vi "PH_SSAC.ProcCases.vi"(0 "i ref in":refnum<vi>, 1 "selector":string, 2 "Data":T1, 3 "call cluster":T2={"Object"="", "Selector"="", "CallType"=enum."synchronous", "Async Object"="", "Async Selector"="", "Data Descriptor"="", "Data"=[], "Error #"=0, "Expire"=0}, 5 "error in (no error)":errorcluster) -> (14 "i ref out":refnum<vi>, 17 "answer cluster":T2={"Object"="", "Selector"="", "CallType"=enum."synchronous", "Async Object"="", "Async Selector"="", "Data Descriptor"="", "Data"=[], "Error #"=0, "Expire"=0}, 19 "error out":errorcluster)   [LabVIEW 2014, in "PH_SSAC.lvlib"]
doc: "This method is called by a process from within the default case in the event loop. The methods of a class that are linked to events will be called from THIS method. Add your code here."
uses:
  PH_SSAC.lvlib
  CS_Core/CSSystem/CoreDefs/CoreDefs.call_type.ctl
  CS_Core/BaseProcess/BaseProcess.descriptor string definition.ctl
  CS_Core/CSSystem/CoreDefs/CoreDefs.rawDataType.ctl
  CS_Core/CSSystem/CoreLib/CoreLib.string 2 byte array.vi
  CS_Core/CSSystem/CoreLib/CoreLib.byte array 2 int.vi
  CS_Core/CSSystem/CoreLib/CoreLib.byte array 2 short.vi
  CS_Core/CSSystem/CoreLib/CoreLib.byte array 2 double.vi
  CS_Core/BaseProcess/BaseProcess.lvlib
  CS_Core/CSSystem/CoreLib/CoreLib.lvlib
  CS_Core/CAEObj/CAEObj.lvlib
  PH_Basics/PH_PSDBWriter/PH_PSDBWriter.lvlib
  PH_Basics/PH_Common/PH_Common.lvlib
  PH_Basics/PH_Img_BaseClass/PH_Img_BaseClass.lvlib
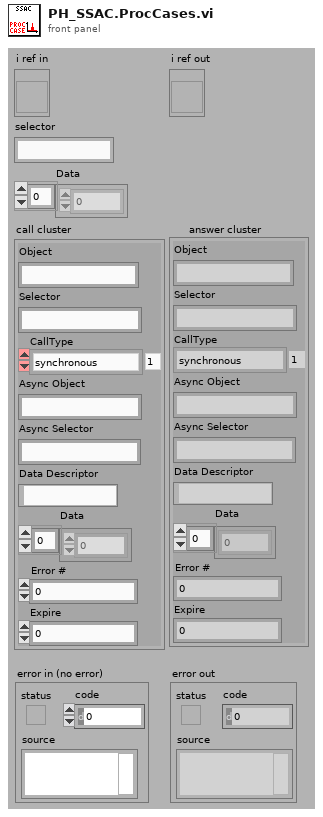
[diagram p1: front panel]
types:
  T1 = typedef "CoreDefs.rawDataType.ctl" = i8[]
  T2 = typedef "CoreDefs.call_type.ctl" = cluster{"Object":string, "Selector":string, "CallType":enum16{"simple", "synchronous", "asynchronous"}, "Async Object":string, "Async Selector":string, "Data Descriptor":T3, "Data":T1, "Error #":i32, "Expire":u32}
  T3 = typedef "BaseProcess.lvlib/BaseProcess.descriptor string definition.ctl" = string
  T4 = typedef "PH_PSDBWriter.lvlib/PH_PSDBWriter.PHELIX-Subsystems.ctl" = i32
  T5 = typedef "PH_SSAC.lvlib/PH_SSAC.i attribute.ctl" = cluster{"GUI Refs":cluster{"Delete":refnum<vi>, "Global On":refnum<vi>, "Cam Source":refnum<vi>, "Frame Main Signal":refnum<vi>, "Frame Background":refnum<vi>, "dt (Gauss smooth)":refnum<vi>, "Calibration Factor":refnum<vi>, "Background acquire":refnum<vi>, "Threshold":refnum<vi>, "Time evolution of mean pulse duration":refnum<vi>, "Mean Pulse Duration":refnum<vi>, "Main signal":refnum<vi>, "Current Pulse Duration":refnum<vi>, "Processed":refnum<vi>, "Saturation":refnum<vi>, "# for Average":refnum<vi>, "Position":refnum<vi>, "BG Status":refnum<vi>, "Save BG data":refnum<vi>, "Read BG Data":refnum<vi>, "Background Calibration Data":refnum<vi>}, "Images":cluster{"OP Image":T6, "GUI Image":T6, "PSDB Image":T6}, "Global On?":bool, "Frame Main":cluster{"x":u32, "dx":u32, "y":u32, "dy":u32}, "Frame Background":cluster{"x":u32, "dx":u32, "y":u32, "dy":u32}, "dt [fs]":dbl, "Calibration Factor [fs/pixel]":dbl, "Threshold":dbl, "Time evolution of mean pulse duration [fs]":dbl[], "Main Signal":cluster{"Time for Main":dbl[], "Signal":dbl[]}, "Processed":bool, "Current Pulse Duration [fs]":dbl, "# for Average":i32, "Position":i32, "Pulse Durations [fs]":dbl[], "BG":cluster{"Acquire?":bool, "Background Calibration Data":T7, "Save Data":bool}}
  T6 = typedef "IMAQ Image.ctl" = refnum<image>
  T7 = typedef "PH_SSAC.lvlib/PH_SSAC.Background Data.ctl" = cluster{"Date":string, "Time":string, "Frame Main":cluster{"x":u32, "dx":u32, "y":u32, "dy":u32}, "dt [fs]":dbl, "Calibration Factor [fs/pixel]":dbl, "Signal":dbl[], "Frame Background":cluster{"x":u32, "dx":u32, "y":u32, "dy":u32}}
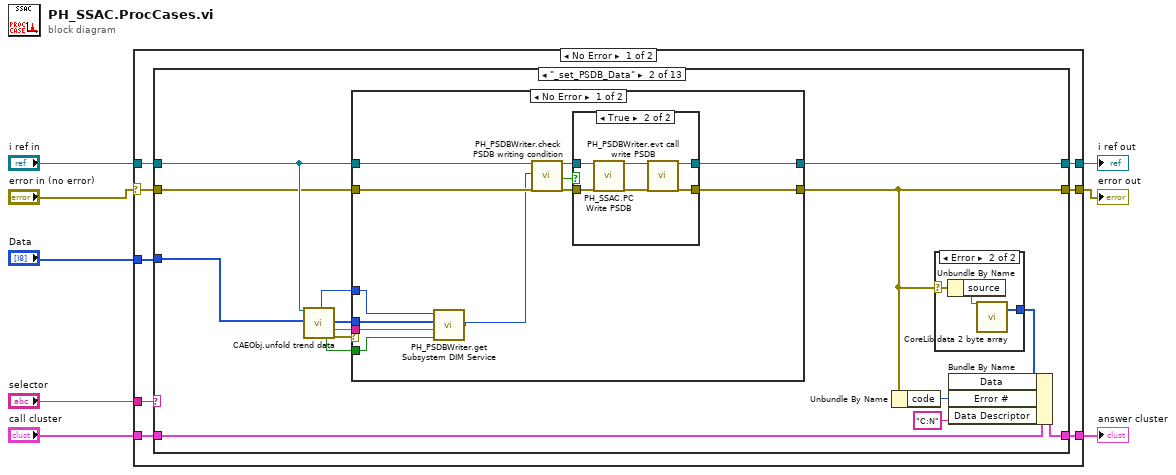
[diagram p0: block diagram]
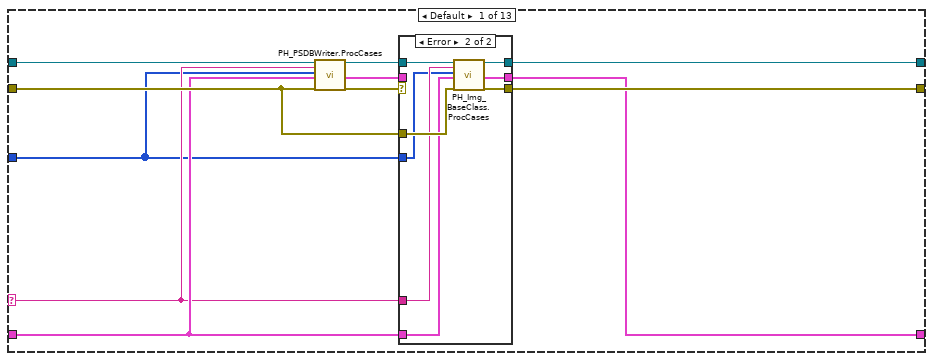
[diagram p2: hidden frame]
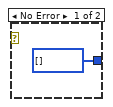
[diagram p6: hidden frame]
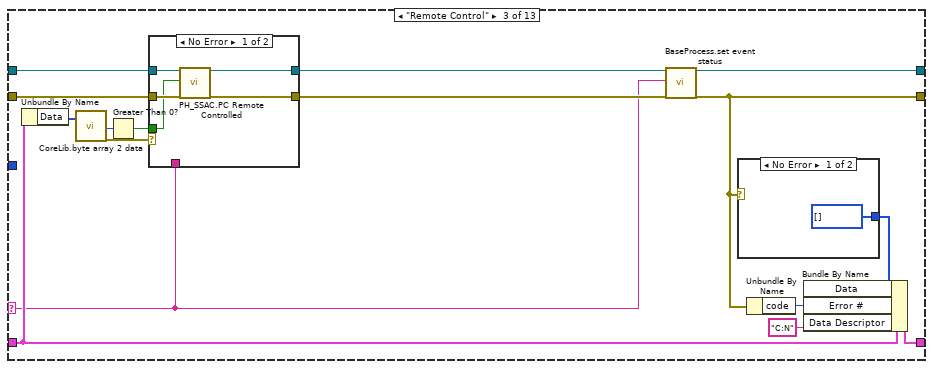
[diagram p7: hidden frame]
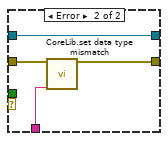
[diagram p8: hidden frame]
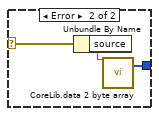
[diagram p9: hidden frame]
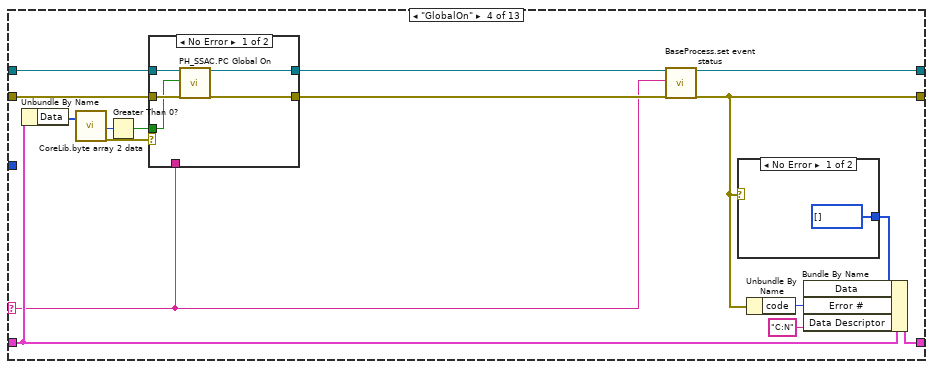
[diagram p10: hidden frame]
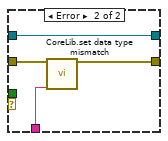
[diagram p11: hidden frame]
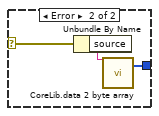
[diagram p12: hidden frame]
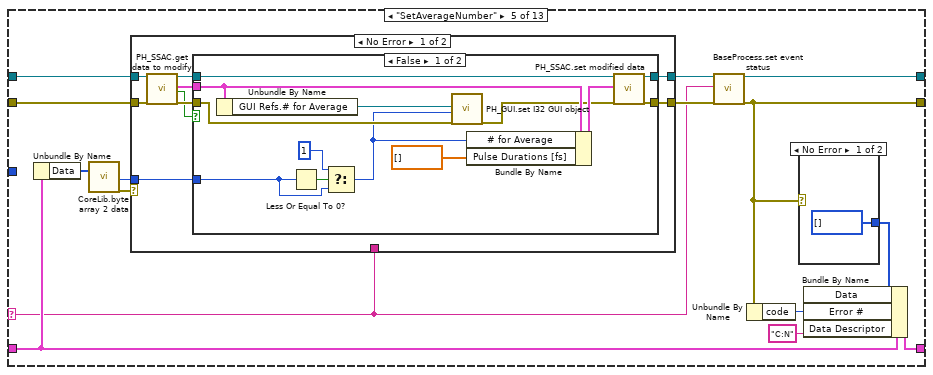
[diagram p13: hidden frame]
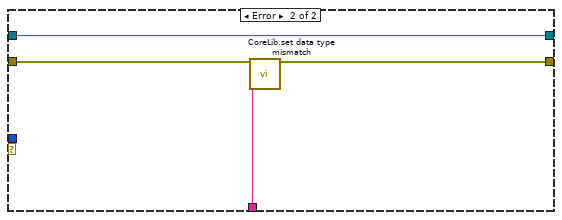
[diagram p15: hidden frame]
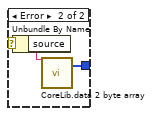
[diagram p16: hidden frame]
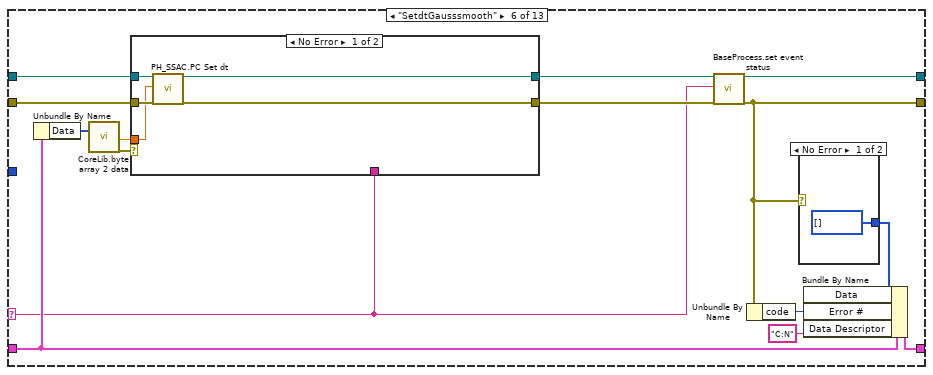
[diagram p17: hidden frame]
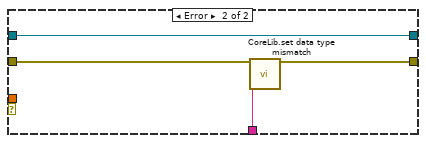
[diagram p18: hidden frame]
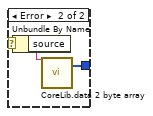
[diagram p19: hidden frame]
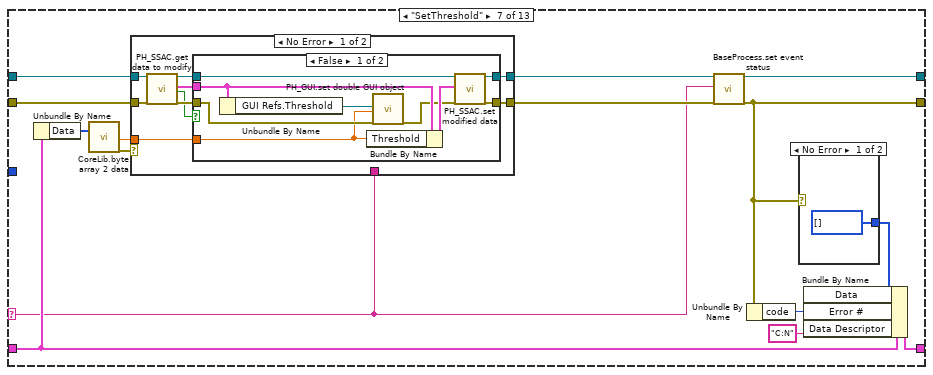
[diagram p20: hidden frame]
diagram:
  n1 = case shown="No Error" "error in (no error)" {
    selector: "error in (no error)" -> [w9 w479]
    tunnel: "selector" -> [w16 _]
    tunnel: [w15 w480] -> w7
    tunnel: "Data" -> [w14 _]
    tunnel: "call cluster" -> [w13 w480]
    tunnel: "i ref in" -> [w12 w481]
    tunnel: [w11 w481] -> w3
    tunnel: [w10 w479] -> w2
    frame No Error {
      n2 = case shown="\"_set_PSDB_Data\"" w16 {
        selector: w16 -> [w18 _ w80 w109 w138 w185 w213 w256 w285 w314 w359 w399 w451]
        tunnel: w14 -> [w17 w39 _ _ _ _ _ _ _ _ _ _ w442]
        tunnel: w12 -> [w27 w43 w84 w113 w143 w190 w218 w261 w290 w319 w364 w404 w444]
        tunnel: [w24 w41 w91 w120 w148 w195 w223 w266 w295 w324 w368 w408 w454] -> w11
        tunnel: w13 -> [w19 w52 w83 w112 w139 w186 w214 w257 w286 w315 w360 w400 w452]
        tunnel: [w21 w51 w94 w123 w151 w198 w226 w269 w298 w327 w371 w411 w457] -> w15
        tunnel: w9 -> [w22 w42 w85 w114 w142 w189 w217 w260 w289 w318 w363 w403 w443]
        tunnel: [w26 w40 w92 w121 w149 w196 w224 w267 w296 w325 w369 w409 w455] -> w10
        frame Default {
          n3 = call "PH_PSDBWriter.ProcCases.vi"("i ref in"=w27, "selector"=w18, "Data"=w17, "call cluster"=w19, "error in"=w22) -> ("i ref out"=w25:refnum<vi>, "answer cluster"=w20:T2, "error out"=w23:errorcluster)  [unwired: 12 in]
          n4 = case shown="Error" w23 {
            selector: w23 -> [w29 _]
            tunnel: [w29 w38] -> w26
            tunnel: w25 -> [w30 w37]
            tunnel: [w30 w36] -> w24
            tunnel: w22 -> [_ w35]
            tunnel: [w28 w34] -> w21
            tunnel: w20 -> [w28 _]
            tunnel: w19 -> [_ w33]
            tunnel: w18 -> [_ w32]
            tunnel: w17 -> [_ w31]
            frame No Error {
            }
            frame Error {
              n5 = call "PH_Img_BaseClass.ProcCases.vi"("i ref in"=w37, "selector"=w32, "Data"=w31, "call cluster"=w33, "error in (no error)"=w35) -> ("i ref out"=w36:refnum<vi>, "answer cluster"=w34:T2, "error out"=w38:errorcluster)  [unwired: 12 in]
            }
          }
        }
        frame "_set_PSDB_Data" {
          n6 = call "CAEObj.unfold trend data.vi"("i ref in"=w43, "raw trend data"=w39) -> ("quality"=w44:i32, "no link"=w47:bool, "data"=w45:i8[], "typeDescriptor"=w46:string, "error out"=w48:errorcluster)  [unwired: 9 in, 4 out]
          n7 = case shown="No Error" w48 {
            tunnel: w42 -> [w65 w75]
            tunnel: [w64 w74] -> w41
            tunnel: [w63 w75] -> w40
            tunnel: w43 -> [w61 w74]
            tunnel: w47 -> [w55 _]
            tunnel: w46 -> [w57 _]
            tunnel: w45 -> [w58 _]
            tunnel: w44 -> [w56 _]
            frame No Error {
              n8 = call "PH_PSDBWriter.get Subsystem DIM Service.vi"("no link"=w55, "typeDescriptor"=w57, "data"=w58, "quality"=w56) -> ("PHELIX Subsystems"=w54:T4)
              n9 = call "PH_PSDBWriter.check PSDB writing condition.vi"("i ref in"=w61, "wanted Subsystem"=w54, "error IO"=w65) -> ("i ref out"=w60:refnum<vi>, "write PSDB?"=w59:bool, "error out"=w62:errorcluster)  [unwired: 14 in]
              n10 = case shown="True" w59 {
                tunnel: w62 -> [w66 w73]
                tunnel: [w67 w70] -> w64
                tunnel: [w66 w68] -> w63
                tunnel: w60 -> [w67 w72]
                frame False {
                }
                frame True {
                  n11 = call "PH_SSAC.PC Write PSDB.vi"("i ref in"=w72, "error IO"=w73) -> ("i ref out"=w71:refnum<vi>, "error out"=w69:errorcluster)  [unwired: 16 in]
                  n12 = call "PH_PSDBWriter.evt call write PSDB.vi"("i ref in"=w71, "error in (no error)"=w69) -> ("i ref out"=w70:refnum<vi>, "error out"=w68:errorcluster)  [unwired: 16 in]
                }
              }
            }
            frame Error {
            }
          }
          n13 = Unbundle By Name(w40) -> ("code"=w53:i32)
          n14 = case shown="Error" w40 {
            selector: w40 -> [_ w79]
            tunnel: [T1 [] ("byteArray out") w78] -> w50
            frame No Error {
            }
            frame Error {
              n15 = Unbundle By Name(w79) -> ("source"=w77:string)
              n16 = call-poly "CoreLib.data 2 byte array.vi"("string"=w77) -> ("byteArray out"=w78:T1)  [unwired: 18 in]
            }
          }
          n17 = Bundle By Name(cluster=w52, "Data"=w50, "Error #"=w53, "Data Descriptor"="C:N") -> (w51:T2)
        }
        frame "Remote Control" {
          n18 = Unbundle By Name(w83) -> ("Data"=w86:T1)
          n19 = call-poly "CoreLib.byte array 2 data.vi"("byteArray"=w86) -> ("i16"=w87:i16, "error out"=w89:errorcluster)  [unwired: 16 in, 1 out]
          n20 = Greater Than 0?(x=w87) -> (x > 0?=w88:bool)
          n21 = case shown="No Error" w89 {
            tunnel: [w97 w104] -> w82
            tunnel: w84 -> [w99 w104]
            tunnel: w85 -> [w98 w103]
            tunnel: [w100 w102] -> w81
            tunnel: w80 -> [_ w101]
            tunnel: w88 -> [w96 _]
            frame No Error {
              n22 = call "PH_SSAC.PC Remote Controlled.vi"("i ref in"=w99, "Remote Controlled?"=w96, "error in (no error)"=w98) -> ("i ref out"=w97:refnum<vi>, "error out"=w100:errorcluster)  [unwired: 15 in]
            }
            frame Error {
              n23 = call "CoreLib.set data type mismatch.vi"("error in (no error)"=w103, "error source"=w101) -> ("error out"=w102:errorcluster)  [unwired: 17 in]
            }
          }
          n24 = call "BaseProcess.set event status.vi"("i ref in"=w82, "EventStatus"=w80, "error in (no error)"=w81) -> ("i ref out"=w91:refnum<vi>, "error out"=w92:errorcluster)  [unwired: 14 in, 1 out]
          n25 = case shown="No Error" w92 {
            selector: w92 -> [_ w108]
            tunnel: [T1 [] ("byteArray out") w107] -> w93
            frame No Error {
            }
            frame Error {
              n26 = Unbundle By Name(w108) -> ("source"=w106:string)
              n27 = call-poly "CoreLib.data 2 byte array.vi"("string"=w106) -> ("byteArray out"=w107:T1)  [unwired: 18 in]
            }
          }
          n28 = Unbundle By Name(w92) -> ("code"=w95:i32)
          n29 = Bundle By Name(cluster=w83, "Data"=w93, "Error #"=w95, "Data Descriptor"="C:N") -> (w94:T2)
        }
        frame "GlobalOn" {
          n30 = Unbundle By Name(w112) -> ("Data"=w115:T1)
          n31 = call-poly "CoreLib.byte array 2 data.vi"("byteArray"=w115) -> ("i16"=w116:i16, "error out"=w118:errorcluster)  [unwired: 16 in, 1 out]
          n32 = Greater Than 0?(x=w116) -> (x > 0?=w117:bool)
          n33 = case shown="No Error" w118 {
            tunnel: [w126 w133] -> w111
            tunnel: w113 -> [w128 w133]
            tunnel: w114 -> [w127 w132]
            tunnel: [w129 w131] -> w110
            tunnel: w109 -> [_ w130]
            tunnel: w117 -> [w125 _]
            frame No Error {
              n34 = call "PH_SSAC.PC Global On.vi"("i ref in"=w128, "Global On?"=w125, "error in (no error)"=w127) -> ("i ref out"=w126:refnum<vi>, "error out"=w129:errorcluster)  [unwired: 15 in]
            }
            frame Error {
              n35 = call "CoreLib.set data type mismatch.vi"("error in (no error)"=w132, "error source"=w130) -> ("error out"=w131:errorcluster)  [unwired: 17 in]
            }
          }
          n36 = call "BaseProcess.set event status.vi"("i ref in"=w111, "EventStatus"=w109, "error in (no error)"=w110) -> ("i ref out"=w120:refnum<vi>, "error out"=w121:errorcluster)  [unwired: 14 in, 1 out]
          n37 = case shown="No Error" w121 {
            selector: w121 -> [_ w137]
            tunnel: [T1 [] ("byteArray out") w136] -> w122
            frame No Error {
            }
            frame Error {
              n38 = Unbundle By Name(w137) -> ("source"=w135:string)
              n39 = call-poly "CoreLib.data 2 byte array.vi"("string"=w135) -> ("byteArray out"=w136:T1)  [unwired: 18 in]
            }
          }
          n40 = Unbundle By Name(w121) -> ("code"=w124:i32)
          n41 = Bundle By Name(cluster=w112, "Data"=w122, "Error #"=w124, "Data Descriptor"="C:N") -> (w123:T2)
        }
        frame "SetAverageNumber" {
          n42 = Unbundle By Name(w139) -> ("Data"=w146:T1)
          n43 = call-poly "CoreLib.byte array 2 data.vi"("byteArray"=w146) -> ("i32"=w144:i32, "error out"=w145:errorcluster)  [unwired: 16 in, 1 out]
          n44 = case shown="No Error" w145 {
            tunnel: [w158 w180] -> w140
            tunnel: w143 -> [w159 w180]
            tunnel: w142 -> [w157 w179]
            tunnel: [w156 w178] -> w141
            tunnel: w144 -> [w153 _]
            tunnel: w138 -> [_ w177]
            frame No Error {
              n45 = call "PH_SSAC.get data to modify.vi"("i ref in"=w159, "error in (no error)"=w157) -> ("i ref out"=w160:refnum<vi>, "i attribute"=w154:T5, "timed out"=w155:bool, "error out"=w161:errorcluster)  [unwired: 14 in]
              n46 = case shown="False" w155 {
                tunnel: w161 -> [w168 w175]
                tunnel: w160 -> [w174 w176]
                tunnel: [w173 w176] -> w158
                tunnel: [w172 w175] -> w156
                tunnel: w154 -> [w170 _]
                tunnel: w153 -> [w163 _]
                frame False {
                  n47 = Unbundle By Name(w170) -> ("GUI Refs.# for Average"=w169:refnum<vi>)
                  n48 = Less Or Equal To 0?(x=w163) -> (x <= 0?=w165:bool)
                  n49 = Select(t=1, s=w165, f=w163) -> (s? t:f=w164:i32)
                  n50 = call "PH_GUI.set I32 GUI object.vi"("I32 GUI Ref"=w169, "value"=w164, "error in (no error)"=w168) -> ("error out"=w167:errorcluster)  [unwired: 16 in]
                  n51 = Bundle By Name(cluster=w170, "# for Average"=w164, "Pulse Durations [fs]"=dbl[] [] ("Average Pulse Duration")) -> (w171:T5)
                  n52 = call "PH_SSAC.set modified data.vi"("i ref in"=w174, "i attribute"=w171, "error in (no error)"=w167) -> ("i ref out"=w173:refnum<vi>, "error out"=w172:errorcluster)  [unwired: 15 in]
                }
                frame True {
                }
              }
            }
            frame Error {
              n53 = call "CoreLib.set data type mismatch.vi"("error in (no error)"=w179, "error source"=w177) -> ("error out"=w178:errorcluster)  [unwired: 17 in]
            }
          }
          n54 = call "BaseProcess.set event status.vi"("i ref in"=w140, "EventStatus"=w138, "error in (no error)"=w141) -> ("i ref out"=w148:refnum<vi>, "error out"=w149:errorcluster)  [unwired: 14 in, 1 out]
          n55 = Unbundle By Name(w149) -> ("code"=w152:i32)
          n56 = case shown="No Error" w149 {
            selector: w149 -> [_ w184]
            tunnel: [T1 [] ("byteArray out") w183] -> w150
            frame No Error {
            }
            frame Error {
              n57 = Unbundle By Name(w184) -> ("source"=w182:string)
              n58 = call-poly "CoreLib.data 2 byte array.vi"("string"=w182) -> ("byteArray out"=w183:T1)  [unwired: 18 in]
            }
          }
          n59 = Bundle By Name(cluster=w139, "Data"=w150, "Error #"=w152, "Data Descriptor"="C:N") -> (w151:T2)
        }
        frame "SetdtGausssmooth" {
          n60 = Unbundle By Name(w186) -> ("Data"=w193:T1)
          n61 = call-poly "CoreLib.byte array 2 data.vi"("byteArray"=w193) -> ("d64"=w191:dbl, "error out"=w192:errorcluster)  [unwired: 16 in, 1 out]
          n62 = case shown="No Error" w192 {
            tunnel: [w203 w208] -> w187
            tunnel: w190 -> [w204 w208]
            tunnel: w189 -> [w202 w207]
            tunnel: [w201 w206] -> w188
            tunnel: w191 -> [w200 _]
            tunnel: w185 -> [_ w205]
            frame No Error {
              n63 = call "PH_SSAC.PC Set dt.vi"("i ref in"=w204, "dt"=w200, "error IO"=w202) -> ("i ref out"=w203:refnum<vi>, "error out"=w201:errorcluster)  [unwired: 15 in]
            }
            frame Error {
              n64 = call "CoreLib.set data type mismatch.vi"("error in (no error)"=w207, "error source"=w205) -> ("error out"=w206:errorcluster)  [unwired: 17 in]
            }
          }
          n65 = call "BaseProcess.set event status.vi"("i ref in"=w187, "EventStatus"=w185, "error in (no error)"=w188) -> ("i ref out"=w195:refnum<vi>, "error out"=w196:errorcluster)  [unwired: 14 in, 1 out]
          n66 = Unbundle By Name(w196) -> ("code"=w199:i32)
          n67 = case shown="No Error" w196 {
            selector: w196 -> [_ w212]
            tunnel: [T1 [] ("byteArray out") w211] -> w197
            frame No Error {
            }
            frame Error {
              n68 = Unbundle By Name(w212) -> ("source"=w210:string)
              n69 = call-poly "CoreLib.data 2 byte array.vi"("string"=w210) -> ("byteArray out"=w211:T1)  [unwired: 18 in]
            }
          }
          n70 = Bundle By Name(cluster=w186, "Data"=w197, "Error #"=w199, "Data Descriptor"="C:N") -> (w198:T2)
        }
        frame "SetThreshold" {
          n71 = Unbundle By Name(w214) -> ("Data"=w221:T1)
          n72 = call-poly "CoreLib.byte array 2 data.vi"("byteArray"=w221) -> ("d64"=w219:dbl, "error out"=w220:errorcluster)  [unwired: 16 in, 1 out]
          n73 = case shown="No Error" w220 {
            tunnel: [w233 w251] -> w215
            tunnel: w218 -> [w234 w251]
            tunnel: w217 -> [w232 w250]
            tunnel: [w231 w249] -> w216
            tunnel: w219 -> [w228 _]
            tunnel: w213 -> [_ w248]
            frame No Error {
              n74 = call "PH_SSAC.get data to modify.vi"("i ref in"=w234, "error in (no error)"=w232) -> ("i ref out"=w235:refnum<vi>, "i attribute"=w229:T5, "timed out"=w230:bool, "error out"=w236:errorcluster)  [unwired: 14 in]
              n75 = case shown="False" w230 {
                tunnel: w236 -> [w239 w246]
                tunnel: w235 -> [w245 w247]
                tunnel: [w244 w247] -> w233
                tunnel: [w243 w246] -> w231
                tunnel: w229 -> [w241 _]
                tunnel: w228 -> [w237 _]
                frame False {
                  n76 = Unbundle By Name(w241) -> ("GUI Refs.Threshold"=w240:refnum<vi>)
                  n77 = Bundle By Name(cluster=w241, "Threshold"=w237) -> (w242:T5)
                  n78 = call "PH_GUI.set double GUI object.vi"("GUI object Ref"=w240, "value"=w237, "error in (no error)"=w239) -> ("error out"=w238:errorcluster)  [unwired: 16 in]
                  n79 = call "PH_SSAC.set modified data.vi"("i ref in"=w245, "i attribute"=w242, "error in (no error)"=w238) -> ("i ref out"=w244:refnum<vi>, "error out"=w243:errorcluster)  [unwired: 15 in]
                }
                frame True {
                }
              }
            }
            frame Error {
              n80 = call "CoreLib.set data type mismatch.vi"("error in (no error)"=w250, "error source"=w248) -> ("error out"=w249:errorcluster)  [unwired: 17 in]
            }
          }
          n81 = call "BaseProcess.set event status.vi"("i ref in"=w215, "EventStatus"=w213, "error in (no error)"=w216) -> ("i ref out"=w223:refnum<vi>, "error out"=w224:errorcluster)  [unwired: 14 in, 1 out]
          n82 = Unbundle By Name(w224) -> ("code"=w227:i32)
          n83 = case shown="No Error" w224 {
            selector: w224 -> [_ w255]
            tunnel: [T1 [] ("byteArray out") w254] -> w225
            frame No Error {
            }
            frame Error {
              n84 = Unbundle By Name(w255) -> ("source"=w253:string)
              n85 = call-poly "CoreLib.data 2 byte array.vi"("string"=w253) -> ("byteArray out"=w254:T1)  [unwired: 18 in]
            }
          }
          n86 = Bundle By Name(cluster=w214, "Data"=w225, "Error #"=w227, "Data Descriptor"="C:N") -> (w226:T2)
        }
        frame "SetCaliFactor" {
          n87 = Unbundle By Name(w257) -> ("Data"=w264:T1)
          n88 = call-poly "CoreLib.byte array 2 data.vi"("byteArray"=w264) -> ("d64"=w262:dbl, "error out"=w263:errorcluster)  [unwired: 16 in, 1 out]
          n89 = case shown="No Error" w263 {
            tunnel: [w274 w279] -> w258
            tunnel: w261 -> [w275 w279]
            tunnel: w260 -> [w273 w278]
            tunnel: [w272 w277] -> w259
            tunnel: w262 -> [w271 _]
            tunnel: w256 -> [_ w276]
            frame No Error {
              n90 = call "PH_SSAC.PC Set Calibration Factor.vi"("i ref in"=w275, "Calibration Factor [fs/pixel]"=w271, "error IO"=w273) -> ("i ref out"=w274:refnum<vi>, "error out"=w272:errorcluster)  [unwired: 15 in]
            }
            frame Error {
              n91 = call "CoreLib.set data type mismatch.vi"("error in (no error)"=w278, "error source"=w276) -> ("error out"=w277:errorcluster)  [unwired: 17 in]
            }
          }
          n92 = call "BaseProcess.set event status.vi"("i ref in"=w258, "EventStatus"=w256, "error in (no error)"=w259) -> ("i ref out"=w266:refnum<vi>, "error out"=w267:errorcluster)  [unwired: 14 in, 1 out]
          n93 = Unbundle By Name(w267) -> ("code"=w270:i32)
          n94 = case shown="No Error" w267 {
            selector: w267 -> [_ w283]
            tunnel: [T1 [] ("byteArray out") w282] -> w268
            frame No Error {
            }
            frame Error {
              n95 = Unbundle By Name(w283) -> ("source"=w281:string)
              n96 = call-poly "CoreLib.data 2 byte array.vi"("string"=w281) -> ("byteArray out"=w282:T1)  [unwired: 18 in]
            }
          }
          n97 = Bundle By Name(cluster=w257, "Data"=w268, "Error #"=w270, "Data Descriptor"="C:N") -> (w269:T2)
        }
        frame "BGAcquire" {
          n98 = Unbundle By Name(w286) -> ("Data"=w293:T1)
          n99 = call-poly "CoreLib.byte array 2 data.vi"("byteArray"=w293) -> ("i16"=w291:i16, "error out"=w292:errorcluster)  [unwired: 16 in, 1 out]
          n100 = Greater Than 0?(x=w291) -> (x > 0?=w284:bool)
          n101 = case shown="No Error" w292 {
            tunnel: [w303 w308] -> w287
            tunnel: w290 -> [w304 w308]
            tunnel: w289 -> [w302 w307]
            tunnel: [w301 w306] -> w288
            tunnel: w284 -> [w300 _]
            tunnel: w285 -> [_ w305]
            frame No Error {
              n102 = call "PH_SSAC.PC Background Acquire.vi"("i ref in"=w304, "BG Acquire"=w300, "error IO"=w302) -> ("i ref out"=w303:refnum<vi>, "error out"=w301:errorcluster)  [unwired: 15 in]
            }
            frame Error {
              n103 = call "CoreLib.set data type mismatch.vi"("error in (no error)"=w307, "error source"=w305) -> ("error out"=w306:errorcluster)  [unwired: 17 in]
            }
          }
          n104 = call "BaseProcess.set event status.vi"("i ref in"=w287, "EventStatus"=w285, "error in (no error)"=w288) -> ("i ref out"=w295:refnum<vi>, "error out"=w296:errorcluster)  [unwired: 14 in, 1 out]
          n105 = Unbundle By Name(w296) -> ("code"=w299:i32)
          n106 = case shown="No Error" w296 {
            selector: w296 -> [_ w312]
            tunnel: [T1 [] ("byteArray out") w311] -> w297
            frame No Error {
            }
            frame Error {
              n107 = Unbundle By Name(w312) -> ("source"=w310:string)
              n108 = call-poly "CoreLib.data 2 byte array.vi"("string"=w310) -> ("byteArray out"=w311:T1)  [unwired: 18 in]
            }
          }
          n109 = Bundle By Name(cluster=w286, "Data"=w297, "Error #"=w299, "Data Descriptor"="C:N") -> (w298:T2)
        }
        frame "BGSave" {
          n110 = Unbundle By Name(w315) -> ("Data"=w322:T1)
          n111 = call-poly "CoreLib.byte array 2 data.vi"("byteArray"=w322) -> ("i16"=w320:i16, "error out"=w321:errorcluster)  [unwired: 16 in, 1 out]
          n112 = Greater Than 0?(x=w320) -> (x > 0?=w313:bool)
          n113 = case shown="No Error" w321 {
            tunnel: [w334 w352] -> w316
            tunnel: w319 -> [w335 w352]
            tunnel: w318 -> [w333 w351]
            tunnel: [w332 w350] -> w317
            tunnel: w313 -> [w329 _]
            tunnel: w314 -> [_ w349]
            frame No Error {
              n114 = call "PH_SSAC.get data to modify.vi"("i ref in"=w335, "error in (no error)"=w333) -> ("i ref out"=w336:refnum<vi>, "i attribute"=w330:T5, "timed out"=w331:bool, "error out"=w337:errorcluster)  [unwired: 14 in]
              n115 = case shown="False" w331 {
                tunnel: w337 -> [w338 w347]
                tunnel: w336 -> [w346 w348]
                tunnel: [w345 w348] -> w334
                tunnel: [w344 w347] -> w332
                tunnel: w330 -> [w342 _]
                tunnel: w329 -> [w339 _]
                frame False {
                  n116 = Unbundle By Name(w342) -> ("GUI Refs.Save BG data"=w341:refnum<vi>)
                  n117 = call "PH_GUI.set boolean GUI object.vi"("Boolean Knob GUI Ref"=w341, "Value"=w339, "error in (no error)"=w338) -> ("error out"=w340:errorcluster)  [unwired: 16 in]
                  n118 = Bundle By Name(cluster=w342, "BG.Save Data"=w339) -> (w343:T5)
                  n119 = call "PH_SSAC.set modified data.vi"("i ref in"=w346, "i attribute"=w343, "error in (no error)"=w340) -> ("i ref out"=w345:refnum<vi>, "error out"=w344:errorcluster)  [unwired: 15 in]
                }
                frame True {
                }
              }
            }
            frame Error {
              n120 = call "CoreLib.set data type mismatch.vi"("error in (no error)"=w351, "error source"=w349) -> ("error out"=w350:errorcluster)  [unwired: 17 in]
            }
          }
          n121 = call "BaseProcess.set event status.vi"("i ref in"=w316, "EventStatus"=w314, "error in (no error)"=w317) -> ("i ref out"=w324:refnum<vi>, "error out"=w325:errorcluster)  [unwired: 14 in, 1 out]
          n122 = Unbundle By Name(w325) -> ("code"=w328:i32)
          n123 = case shown="No Error" w325 {
            selector: w325 -> [_ w356]
            tunnel: [T1 [] ("byteArray out") w355] -> w326
            frame No Error {
            }
            frame Error {
              n124 = Unbundle By Name(w356) -> ("source"=w354:string)
              n125 = call-poly "CoreLib.data 2 byte array.vi"("string"=w354) -> ("byteArray out"=w355:T1)  [unwired: 18 in]
            }
          }
          n126 = Bundle By Name(cluster=w315, "Data"=w326, "Error #"=w328, "Data Descriptor"="C:N") -> (w327:T2)
        }
        frame "BGRead" {
          n127 = Unbundle By Name(w360) -> ("Data"=w366:T1)
          n128 = call-poly "CoreLib.byte array 2 data.vi"("byteArray"=w366) -> ("i16"=w365:i16, "error out"=w357:errorcluster)  [unwired: 16 in, 1 out]
          n129 = Greater Than 0?(x=w365) -> (x > 0?=w358:bool)
          n130 = case shown="No Error" w357 {
            tunnel: w364 -> [w377 w378]
            tunnel: w363 -> [w375 w381]
            tunnel: [w374 w380] -> w362
            tunnel: [w376 w378] -> w361
            tunnel: w359 -> [_ w379]
            tunnel: w358 -> [w373 _]
            frame No Error {
              n131 = call "PH_SSAC.PC Background Read.vi"("i ref in"=w377, "BG Read"=w373, "error IO"=w375) -> ("i ref in"=w376:refnum<vi>, "error out"=w374:errorcluster)  [unwired: 15 in]
            }
            frame Error {
              n132 = call "CoreLib.set data type mismatch.vi"("error in (no error)"=w381, "error source"=w379) -> ("error out"=w380:errorcluster)  [unwired: 17 in]
            }
          }
          n133 = call "BaseProcess.set event status.vi"("i ref in"=w361, "EventStatus"=w359, "error in (no error)"=w362) -> ("i ref out"=w368:refnum<vi>, "error out"=w369:errorcluster)  [unwired: 14 in, 1 out]
          n134 = Unbundle By Name(w369) -> ("code"=w372:i32)
          n135 = case shown="No Error" w369 {
            selector: w369 -> [_ w385]
            tunnel: [T1 [] ("byteArray out") w384] -> w370
            frame No Error {
            }
            frame Error {
              n136 = Unbundle By Name(w385) -> ("source"=w383:string)
              n137 = call-poly "CoreLib.data 2 byte array.vi"("string"=w383) -> ("byteArray out"=w384:T1)  [unwired: 18 in]
            }
          }
          n138 = Bundle By Name(cluster=w360, "Data"=w370, "Error #"=w372, "Data Descriptor"="C:N") -> (w371:T2)
        }
        frame "SetFrame" {
          n139 = Unbundle By Name(w400) -> ("Data"=w406:T1)
          n140 = call-poly "CoreLib.byte array 2 data.vi"("byteArray"=w406) -> ("byteArray out"=w393:T1, "i32"=w405:i32, "error out"=w395:errorcluster)  [unwired: 16 in]
          n141 = call-poly "CoreLib.byte array 2 data.vi"("byteArray"=w393, "error in (no error)"=w395) -> ("byteArray out"=w392:T1, "i32"=w389:i32, "error out"=w398:errorcluster)  [unwired: 15 in]
          n142 = call-poly "CoreLib.byte array 2 data.vi"("byteArray"=w392, "error in (no error)"=w398) -> ("byteArray out"=w391:T1, "i32"=w388:i32, "error out"=w397:errorcluster)  [unwired: 15 in]
          n143 = call-poly "CoreLib.byte array 2 data.vi"("byteArray"=w391, "error in (no error)"=w397) -> ("byteArray out"=w390:T1, "i32"=w387:i32, "error out"=w396:errorcluster)  [unwired: 15 in]
          n144 = call-poly "CoreLib.byte array 2 data.vi"("byteArray"=w390, "error in (no error)"=w396) -> ("i32"=w386:i32, "error out"=w394:errorcluster)  [unwired: 15 in, 1 out]
          n145 = case shown="No Error" w394 {
            tunnel: [w432 w437] -> w401
            tunnel: w404 -> [w433 w437]
            tunnel: w403 -> [w431 w436]
            tunnel: [w430 w435] -> w402
            tunnel: w405 -> [w421 _]
            tunnel: w399 -> [_ w434]
            tunnel: w389 -> [w428 _]
            tunnel: w388 -> [w427 _]
            tunnel: w387 -> [w426 _]
            tunnel: w386 -> [w425 _]
            frame No Error {
              n146 = To Unsigned Long Integer(number=w428) -> (unsigned 32bit integer=w423:u32)
              n147 = To Unsigned Long Integer(number=w427) -> (unsigned 32bit integer=w418:u32)
              n148 = To Unsigned Long Integer(number=w426) -> (unsigned 32bit integer=w422:u32)
              n149 = To Unsigned Long Integer(number=w425) -> (unsigned 32bit integer=w413:u32)
              n150 = Equal To 0?(x=w418) -> (x = 0?=w420:bool)
              n151 = Equal To 0?(x=w413) -> (x = 0?=w416:bool)
              n152 = Select(t=u32 1, s=w420, f=w418) -> (s? t:f=w419:u32)
              n153 = Select(t=u32 1, s=w416, f=w413) -> (s? t:f=w414:u32)
              n154 = Bundle By Name(cluster=cluster{"x":u32, "dx":u32, "y":u32, "dy":u32} {"x"=0, "dx"=0, "y"=0, "dy"=0} ("Frame"), "x"=w423, "dx"=w419, "y"=w422, "dy"=w414) -> (w424:cluster{"x":u32, "dx":u32, "y":u32, "dy":u32})
              n155 = call "PH_SSAC.PC Set Frame.vi"("i ref in"=w433, "Signal"=w421, "Frame"=w424, "error IO"=w431) -> ("i ref out"=w432:refnum<vi>, "error out"=w430:errorcluster)  [unwired: 14 in]
            }
            frame Error {
              n156 = call "CoreLib.set data type mismatch.vi"("error in (no error)"=w436, "error source"=w434) -> ("error out"=w435:errorcluster)  [unwired: 17 in]
            }
          }
          n157 = call "BaseProcess.set event status.vi"("i ref in"=w401, "EventStatus"=w399, "error in (no error)"=w402) -> ("i ref out"=w408:refnum<vi>, "error out"=w409:errorcluster)  [unwired: 14 in, 1 out]
          n158 = Unbundle By Name(w409) -> ("code"=w412:i32)
          n159 = case shown="No Error" w409 {
            selector: w409 -> [_ w441]
            tunnel: [T1 [] ("byteArray out") w440] -> w410
            frame No Error {
            }
            frame Error {
              n160 = Unbundle By Name(w441) -> ("source"=w439:string)
              n161 = call-poly "CoreLib.data 2 byte array.vi"("string"=w439) -> ("byteArray out"=w440:T1)  [unwired: 18 in]
            }
          }
          n162 = Bundle By Name(cluster=w400, "Data"=w410, "Error #"=w412, "Data Descriptor"="C:N") -> (w411:T2)
        }
        frame "_Camlinked" {
          n163 = call "CAEObj.unfold trend data.vi"("i ref in"=w444, "raw trend data"=w442) -> ("no link"=w448:bool, "data"=w447:i8[], "typeDescriptor"=w449:string, "error out"=w450:errorcluster)  [unwired: 9 in, 5 out]
          n164 = case shown="No Error" w450 {
            tunnel: [w462 w474] -> w445
            tunnel: w444 -> [w465 w474]
            tunnel: w443 -> [w464 w473]
            tunnel: [w460 w473] -> w446
            tunnel: w449 -> [_ _]
            tunnel: w448 -> [w459 _]
            tunnel: w447 -> [_ _]
            frame No Error {
              n165 = call "PH_SSAC._PC Cam linked.vi"("i ref in"=w465, "cam not linked?"=w459, "error IO"=w464) -> ("i ref out"=w463:refnum<vi>, "error out"=w461:errorcluster)  [unwired: 15 in]
              n166 = case shown="True" w459 {
                tunnel: w463 -> [w467 w472]
                tunnel: [w467 w471] -> w462
                tunnel: [w466 w470] -> w460
                tunnel: w461 -> [w466 w469]
                frame False {
                }
                frame True {
                  n167 = call "PH_SSAC.PC Global On.vi"("i ref in"=w472, "Global On?"=FALSE, "error in (no error)"=w469) -> ("i ref out"=w471:refnum<vi>, "error out"=w470:errorcluster)  [unwired: 15 in]
                }
              }
            }
            frame Error {
            }
          }
          n168 = call "BaseProcess.set event status.vi"("i ref in"=w445, "EventStatus"=w451, "error in (no error)"=w446) -> ("i ref out"=w454:refnum<vi>, "error out"=w455:errorcluster)  [unwired: 14 in, 1 out]
          n169 = case shown="No Error" w455 {
            selector: w455 -> [_ w478]
            tunnel: [T1 [] ("byteArray out") w477] -> w456
            frame No Error {
            }
            frame Error {
              n170 = Unbundle By Name(w478) -> ("source"=w476:string)
              n171 = call-poly "CoreLib.data 2 byte array.vi"("string"=w476) -> ("byteArray out"=w477:T1)  [unwired: 18 in]
            }
          }
          n172 = Unbundle By Name(w455) -> ("code"=w458:i32)
          n173 = Bundle By Name(cluster=w452, "Data"=w456, "Error #"=w458, "Data Descriptor"="C:N") -> (w457:T2)
        }
      }
    }
    frame Error {
    }
  }
  "answer cluster" <- w7
  "i ref out" <- w3
  "error out" <- w2
